vi "FilterDeviceStartList_ForAlreadyOpen.vi"(9 "Input Device Names":string[](array[string]), 11 "All Devices Core Info":string[][](array[string])) -> (1 "Output Filtered Device Array":string[](array[string]))   [LabVIEW 2020]
uses:
  <userlib>/_OpenG.lib/array/array.llb/Filter 1D Array (String)__ogtk.vi
  <userlib>/_OpenG.lib/array/array.llb/Empty 1D Array (I32)__ogtk.vi
panel:
  out "All Open Devices":string[](array[string])
  out "Open Devices":string[](array[string])
  out "IP Addresses":string[](array[string])
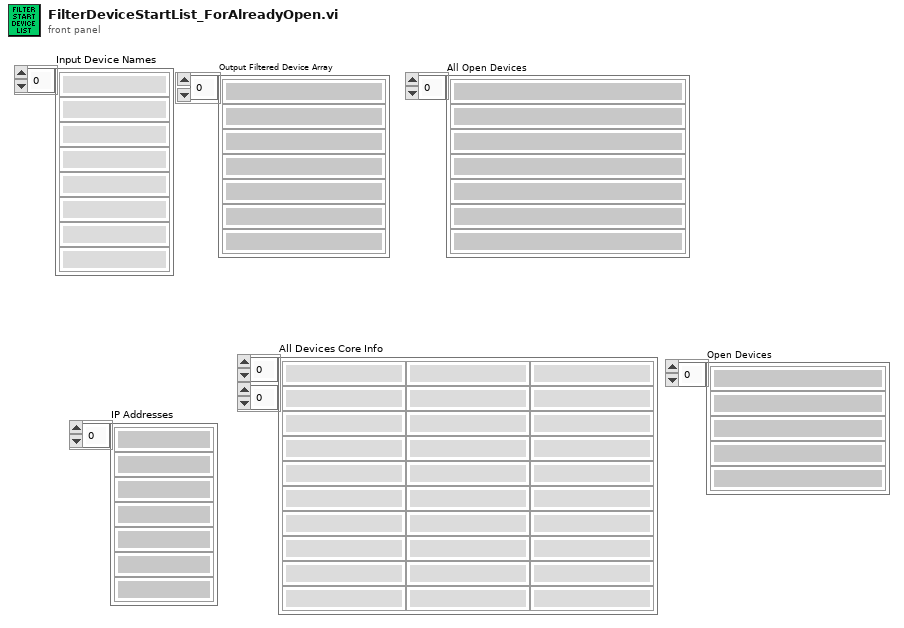
[diagram p1: front panel]
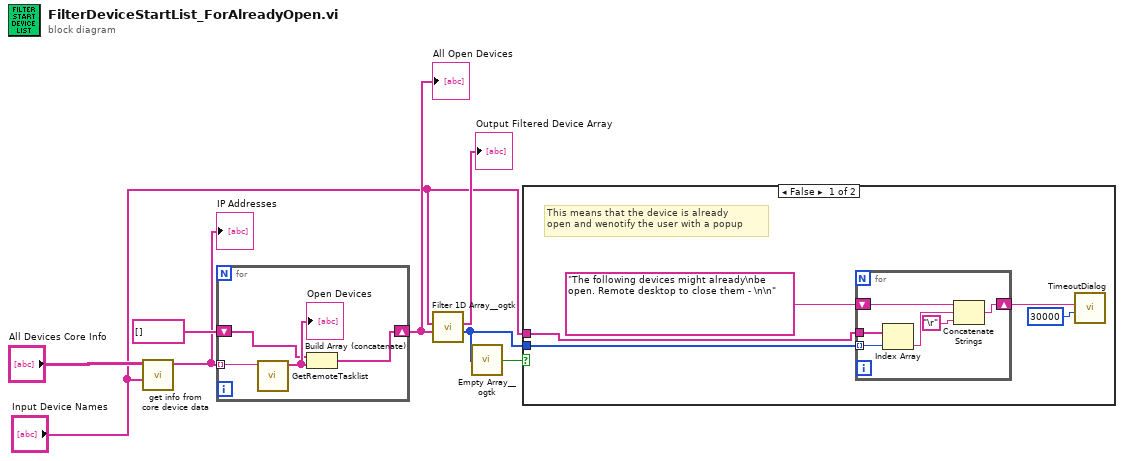
[diagram p0: block diagram]
diagram:
  n1 = call "get info from core device data.vi"("devices to get data from"="Input Device Names", "All Devices Core Info"="All Devices Core Info") -> ("IP Addresses"=w1:string[])  [unwired: 2 in, 3 out]
  "IP Addresses" <- w1
  n2 = for {
    tunnel: w1 -> [w12] mode=indexing
    shift-right: [w9] -> w6
    shift-left: string[] [] -> [w10]
    n3 = call "GetRemoteTasklist.vi"("Input IP Address"=w12) -> ("Open Devices"=w11:string[])  [unwired: 8 in, 2 out]
    "Open Devices" <- w11
    n4 = Build Array (concatenate)(w10, w11) -> (w9:string[])
  }
  "All Open Devices" <- w6
  n5 = call-poly <userlib>:"Filter 1D Array__ogtk.vi"("items to filter"=w6, "array"="Input Device Names") -> ("filtered item indices"=w3:i32[], "filtered array"=→"Output Filtered Device Array":string[])  [unwired: 4 in]
  n6 = call-poly <userlib>:"Empty Array__ogtk.vi"("Array"=w3) -> ("Empty Array?"=w5:bool)  [unwired: 8 in]
  n7 = case shown="False" w5 {
    tunnel: w3 -> [w17 _]
    tunnel: "Input Device Names" -> [w16 _]
    frame False {
      # "This means that the device is already \nopen and wenotify the user with a popup"
      n8 = for {
        tunnel: w17 -> [w22] mode=indexing
        tunnel: w16 -> [w23]
        shift-right: [w21] -> w15
        shift-left: "The following devices might already\nbe open. Remote desktop to close them - \n\n" -> [w20]
        n9 = Index Array(array=w23, index=w22) -> (element=w19:string)
        n10 = Concatenate Strings(w20, w19, "\r") -> (w21:string)
      }
      n11 = call "TimeoutDialog.vi"("message 2"=w15, "Timeout(ms)"=u32 30000) -> ()  [unwired: 9 in]
    }
    frame True {
      # "This means that the device we want \nto open is not already open"
    }
  }
